vi "Parse from String.vi"(8 "error in (no error)":errorcluster, 10 "JSON String":string) -> (0 "error out":errorcluster, 3 "JSON out":refnum<class "JSON Null.lvclass">)   [LabVIEW 2015]
uses:
  JSON Datatype/JSON Null.lvclass
  JSON Helper.lvclass
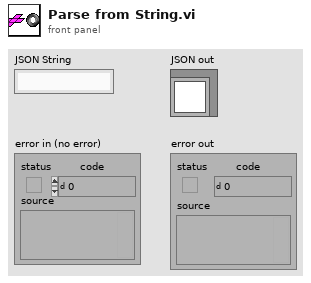
[diagram p1: front panel]
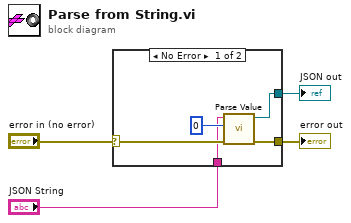
[diagram p0: block diagram]
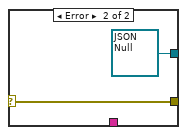
[diagram p2: hidden frame]
diagram:
  n1 = case shown="No Error" "error in (no error)" {
    selector: "error in (no error)" -> [w8 w11]
    tunnel: [w6 w11] -> w3
    tunnel: [w7 refnum<class "JSON Null.lvclass"> refnum ("LVJSON.lvlib:JSON Null.lvclass")] -> w2
    tunnel: "JSON String" -> [w5 _]
    frame No Error {
      n2 = call "Parse Value.vi"("error in (no error)"=w8, "Index In"=0, "JSON String"=w5) -> ("error out"=w6:errorcluster, "JSON out"=w7:refnum<class "JSON Null.lvclass">)  [unwired: 6 in, 1 out]
    }
    frame Error {
    }
  }
  "error out" <- w3
  "JSON out" <- w2
